vi "Less Than.vi"(1 "y":refnum<class "People By Name Wrapper.lvclass">, 2 "x":refnum<class "People By Name Wrapper.lvclass">) -> (0 "less than?":bool)   [LabVIEW 2023, in "People By Name Wrapper.lvclass"]
doc: "Returns TRUE if the value of <b>x</b> is less than the value of <b>y</b>."
uses:
  People By Name Wrapper.lvclass
  People By Name Wrapper.lvclass/People By Name Wrapper.ctl
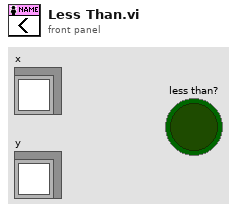
[diagram p1: front panel]
types:
  T1 = typedef "Person Information.ctl" = cluster{"ID":u32, "Family Name":string, "Given Name":string, "Birth Date":timestamp}
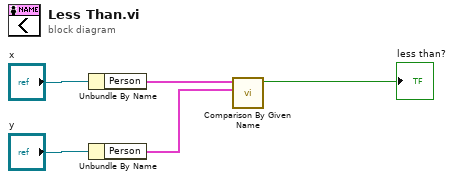
[diagram p0: block diagram]
diagram:
  n1 = Unbundle By Name("x") -> ("Person"=w3:T1)
  n2 = Unbundle By Name("y") -> ("Person"=w2:T1)
  n3 = call "Comparison By Given Name.vi"("Person B"=w2, "Person A"=w3) -> ("Swap?"=→"less than?":bool)  [unwired: 9 in]
